vi "SyntaxOperation.vi"(8 "error in (no error)":errorcluster, 11 "Parsed Expression In":T1) -> (0 "error out":errorcluster, 1 "Error Index Out":i32, 2 "Token":string[](array[string]), 3 "Parsed Expression Out":T1)   [LabVIEW 2014, in "MathProg.lvlib"]
uses:
  MathProg.lvlib
  TypeDefs/ParsedExpression.ctl
  TypeDefs/typeMed.ctl
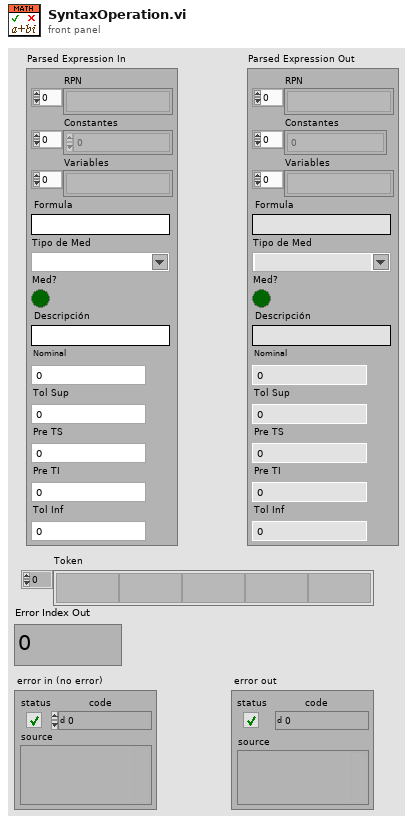
[diagram p1: front panel]
types:
  T1 = typedef "MathProg.lvlib/ParsedExpression.ctl" = cluster{"RPN ":string[], "Constantes":sgl[], "Variables":string[], "Formula":string, "Tipo de Med":T2, "Med?":bool, "Descripción":string, "Nominal":sgl, "Tol Sup":sgl, "Pre TS":sgl, "Pre TI":sgl, "Tol Inf":sgl}
  T2 = typedef "MathProg.lvlib/typeMed.ctl" = string
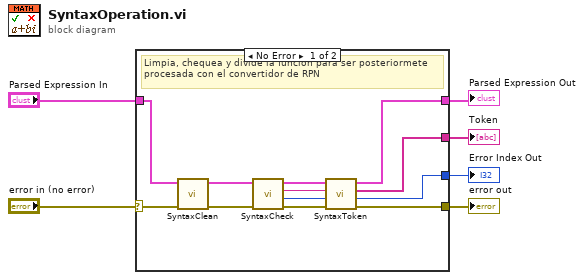
[diagram p0: block diagram]
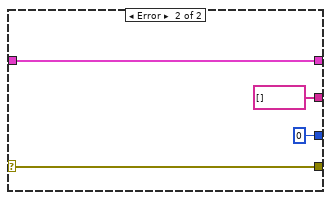
[diagram p2: hidden frame]
diagram:
  n1 = case shown="No Error" "error in (no error)" {
    selector: "error in (no error)" -> [w12 w21]
    tunnel: [w11 w21] -> w6
    tunnel: "Parsed Expression In" -> [w10 w22]
    tunnel: [w9 w22] -> w2
    tunnel: [w8 string[] [] ("Token")] -> w4
    tunnel: [w7 0 ("Error Index Out")] -> w3
    frame No Error {
      # "Limpia, chequea y divide la función para ser posteriormete procesada con el convertidor de RPN"
      n2 = call "SyntaxClean.vi"("error in (no error)"=w12, "Parsed Expression In"=w10) -> ("error out"=w16:errorcluster, "Parsed Expression Out"=w17:T1)  [unwired: 8 in]
      n3 = call "SyntaxCheck.vi"("error in"=w16, "Parsed Expression In"=w17) -> ("error out"=w13:errorcluster, "Error Index"=w14:i32, "Funcion Analizada"=w15:string, "Parsed Expression Out"=w18:T1)  [unwired: 6 in]
      n4 = call "SyntaxToken.vi"("error in"=w13, "Error Index In"=w14, "Funcion Analizada"=w15, "Parsed Expression In"=w18) -> ("error out"=w11:errorcluster, "Error Index Out"=w7:i32, "Token"=w8:string[], "Parsed Expression Out"=w9:T1)  [unwired: 4 in]
    }
    frame Error {
    }
  }
  "error out" <- w6
  "Error Index Out" <- w3
  "Token" <- w4
  "Parsed Expression Out" <- w2
